vi "Create Greyscale Test Image.vi"(8 "error in (no error)":errorcluster, 11 "Preallocated Image Size":T1) -> (0 "error out":errorcluster, 2 "GreyscaleImage":u8[][](array[numeric]), 3 "Data Value Reference out":refnum<data-value>)   [LabVIEW 2020, in "g_ar_toolkit.test.lvlib" / "Image.lvclass"]
uses:
  g_ar_toolkit.test/Image/Image.lvclass
  g_ar_toolkit.test/Image/Image.lvclass/Image.ctl
  g_ar_toolkit.image.lvlib
  CreateEmptyImageGreyscale.vi
  Image Size (Fixed).ctl
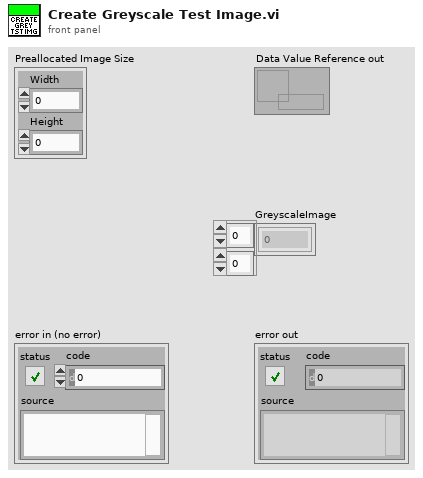
[diagram p1: front panel]
types:
  T1 = typedef "g_ar_toolkit.image.lvlib/Image Size (Fixed).ctl" = cluster{"Width":u16, "Height":u16}
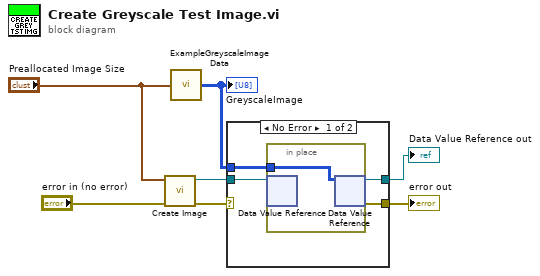
[diagram p0: block diagram]
diagram:
  n1 = call-poly "Create Image.vi"("error in (no error)"="error in (no error)", "Preallocated Image Size (Default 0,0)"="Preallocated Image Size") -> ("error out"=w4:errorcluster, "New Greyscale Image"=w3:refnum<data-value>)  [unwired: 8 in]
  n2 = call "ExampleGreyscaleImageData.vi"("Image Size"="Preallocated Image Size") -> ("GreyscaleImage"=w6:u8[][])
  "GreyscaleImage" <- w6
  n3 = case shown="No Error" w4 {
    selector: w4 -> [_ w13]
    tunnel: w3 -> [w11 w14]
    tunnel: [w10 w14] -> w7
    tunnel: [w9 w13] -> w5
    tunnel: w6 -> [w8 _]
    frame No Error {
      n4 = in-place {
        in-place-border: w8 -> [w12]
        n5 = in-place-dvr #1(w11) -> ()  [unwired: 2 out]
        n6 = in-place-dvr #1(w12) -> (w10:refnum<data-value>, w9:errorcluster)
      }
    }
    frame Error {
    }
  }
  "Data Value Reference out" <- w7
  "error out" <- w5
